vi "Hat Switch Interpreter.vi"(5 "Axis 6":dbl, 6 "Axis 5":dbl) -> (0 "Buttons":bool[](array[boolean]), 1 "Buttons Pressed":bool[](array[boolean]), 2 "Enum Status":T2(ring), 3 "Numeric Status":u8, 4 "Hat Switch Cluster":T1)   [LabVIEW 2013]
panel:
  # "ENUM LAYOUT"
  # "NUMERIC LAYOUT"
  # "North"
  # "1"
  # "Northeast"
  # "2"
  # "Northwest"
  # "8"
  # "West"
  # "East"
  # "7"
  # "3"
  # "Null"
  # "0"
  # "Southwest"
  # "Southeast"
  # "6"
  # "4"
  # "5"
  # "South"
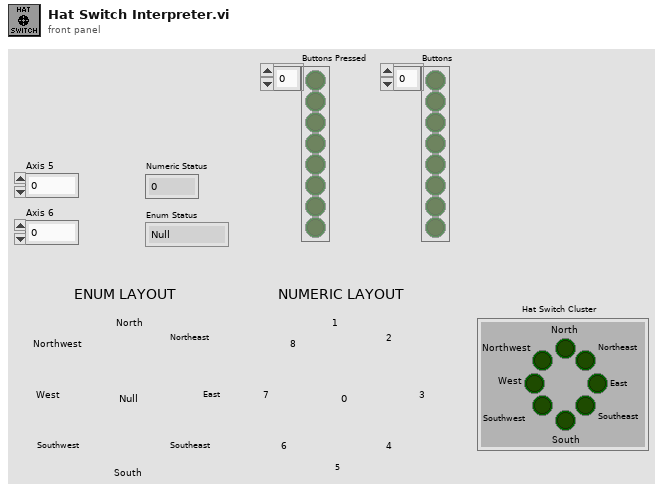
[diagram p1: front panel]
types:
  T1 = cluster{"North":bool, "Northeast":bool, "East":bool, "Southeast":bool, "South":bool, "Southwest":bool, "West":bool, "Northwest":bool}
  T2 = enum8{"Null", "North", "Northeast", "East", "Southeast", "South", "Southwest", "West", "Northwest"}
  T3 = cluster{"North":bool, "Northeast":bool, "East":bool, "Southeast":bool, "South":bool, "Northwest":bool, "Southwest":bool, "West":bool}
  T4 = cluster{"[0]":bool, "[1]":bool, "[2]":bool, "[3]":bool, "[4]":bool, "[5]":bool, "[6]":bool, "[7]":bool, "[8]":bool}
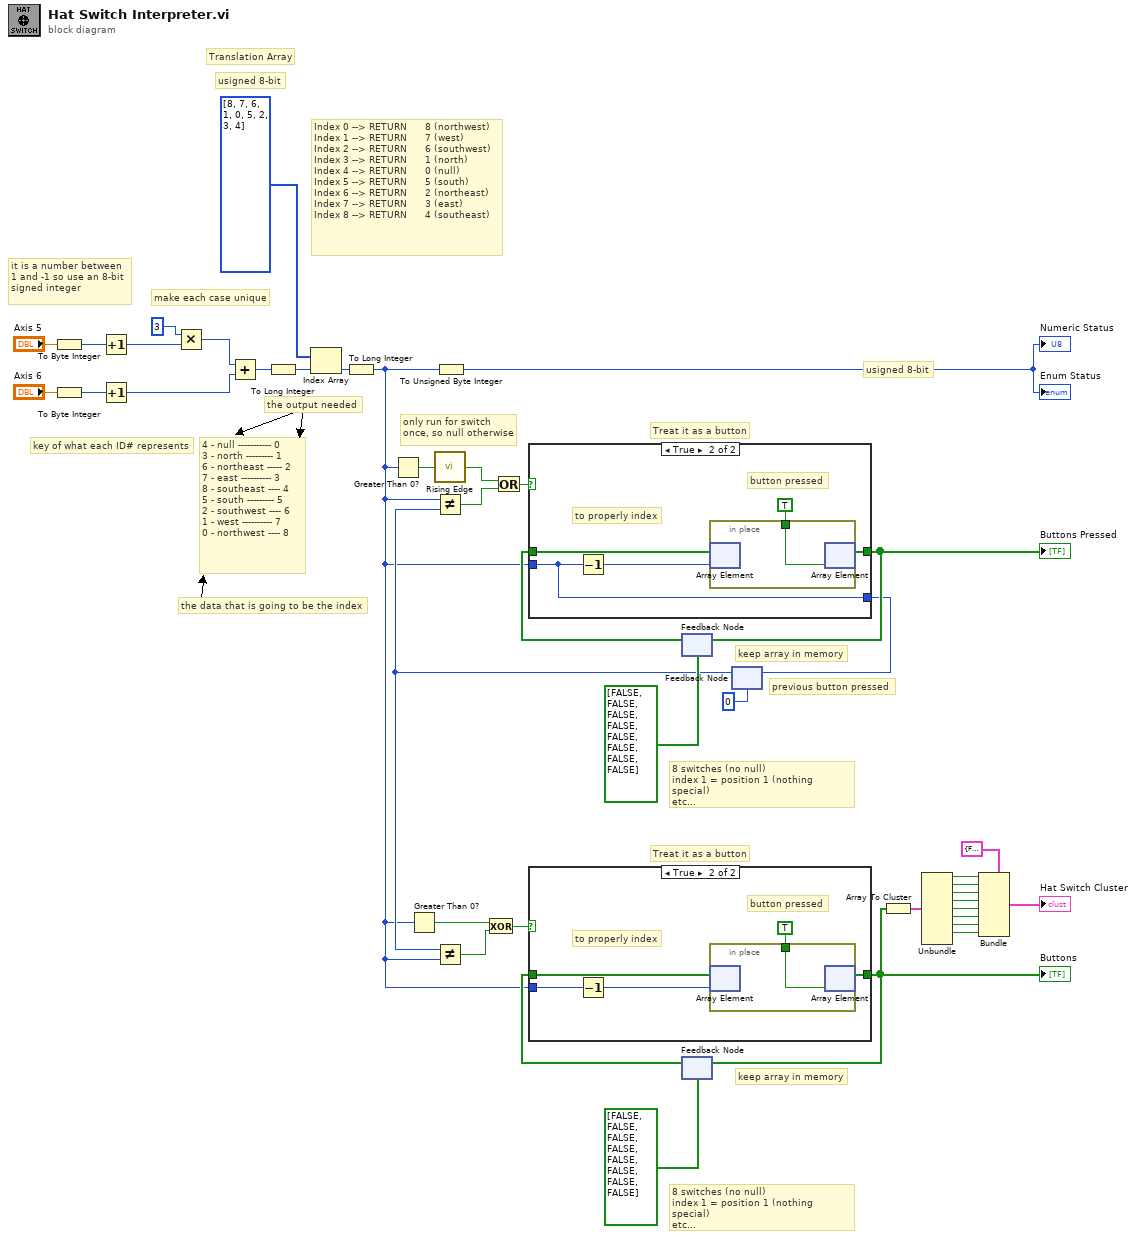
[diagram p0: block diagram]
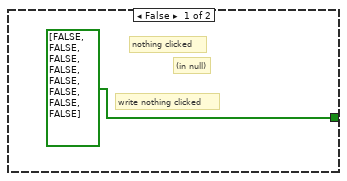
[diagram p2: hidden frame]
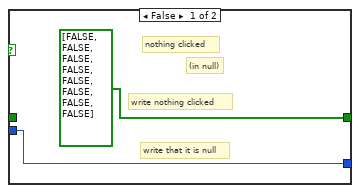
[diagram p3: hidden frame]
diagram:
  # "keep array in memory"
  # "8 switches (no null)\nindex 1 = position 1 (nothing special)\netc..."
  # "Treat it as a button"
  # "only run for switch\nonce, so null otherwise"
  # "keep array in memory"
  # "previous button pressed"
  # "8 switches (no null)\nindex 1 = position 1 (nothing special)\netc..."
  # "Treat it as a button"
  # "usigned 8-bit"
  # "the data that is going to be the index"
  # "the output needed"
  # "key of what each ID# represents"
  # "Index 0 --> RETURN      8 (northwest)\nIndex 1 --> RETURN      7 (west)\nIndex 2 --> RETURN      6 (southwest)\nIndex 3 --> RETURN      1 (north)\nIndex 4 --> RETURN      0 (null)\nIndex 5 --> RETURN      5 (south)\nIndex 6 --> RETURN      2 (northeast)\nIndex 7 --> RETURN      3 (east)\nIndex 8 --> RETURN      4 (southeast)"
  # "4 - null ----------- 0\n3 - north --------- 1\n6 - northeast ----- 2\n7 - east ---------- 3\n8 - southeast ---- 4\n5 - south --------- 5\n2 - southwest ---- 6\n1 - west ---------- 7\n0 - northwest ---- 8"
  # "Translation Array"
  # "usigned 8-bit"
  # "it is a number between\n1 and -1 so use an 8-bit\nsigned integer"
  # "make each case unique"
  n1 = To Byte Integer(number="Axis 5") -> (8bit integer=w35:i8)
  n2 = To Byte Integer(number="Axis 6") -> (8bit integer=w34:i8)
  n3 = Increment(x=w35) -> (x+1=w39:i8)
  n4 = Increment(x=w34) -> (x+1=w36:i8)
  n5 = Multiply(x=i8 3, y=w39) -> (x*y=w37:i8)
  n6 = Add(x=w37, y=w36) -> (x+y=w32:i8)
  n7 = To Long Integer(number=w32) -> (32bit integer=w31:i32)
  n8 = Index Array(array=u8[] [8, 7, 6, 1, 0, 5, 2, 3, 4], index=w31) -> (element=w22:u8)
  n9 = To Long Integer(number=w22) -> (32bit integer=w15:i32)
  n10 = Greater Than 0?(x=w15) -> (x > 0?=w25:bool)
  n11 = Greater Than 0?(x=w15) -> (x > 0?=w17:bool)
  n12 = call "Rising Edge.vi"("Input"=w25) -> ("Rising Edge"=w24:bool)
  n13 = To Unsigned Byte Integer(number=w15) -> (unsigned 8bit integer=→"Numeric Status" →"Enum Status":u8)
  n14 = feedback #1(bool[] [FALSE, FALSE, FALSE, FALSE, FALSE, FALSE, FALSE, FALSE]) -> (w29:bool[])
  n15 = feedback #2(bool[] [FALSE, FALSE, FALSE, FALSE, FALSE, FALSE, FALSE, FALSE]) -> (w19:bool[])
  n16 = feedback #3(0) -> (w16:i32)
  n17 = Not Equal?(x=w15, y=w16) -> (x != y?=w21:bool)
  n18 = Not Equal?(x=w16, y=w15) -> (x != y?=w13:bool)
  n19 = Exclusive Or(1:w13, 2:w17) -> (0:w14:bool)
  n20 = Or(x=w24, y=w21) -> (x .or. y?=w23:bool)
  n21 = case shown="True" w23 {
    tunnel: w29 -> [_ w48]
    tunnel: [bool[] [FALSE, FALSE, FALSE, FALSE, FALSE, FALSE, FALSE, FALSE] w47] -> w28
    tunnel: w15 -> [w43 w44]
    tunnel: [w43 w44] -> w26
    frame False {
      # "write nothing clicked"
      # "write that it is null"
      # "(in null)"
      # "nothing clicked"
    }
    frame True {
      # "to properly index"
      # "button pressed"
      n22 = Decrement(x=w44) -> (x-1=w45:i32)
      n23 = in-place {
        in-place-border: TRUE -> [w49]
        n24 = in-place-array #4(w48, w45) -> ()  [unwired: 1 out]
        n25 = in-place-array #4(w49) -> (w47:bool[])  [unwired: 1 out]
      }
    }
  }
  "Buttons Pressed" <- w28
  n26 = case shown="True" w14 {
    tunnel: w19 -> [_ w55]
    tunnel: [bool[] [FALSE, FALSE, FALSE, FALSE, FALSE, FALSE, FALSE, FALSE] w54] -> w12
    tunnel: w15 -> [_ w51]
    frame False {
      # "write nothing clicked"
      # "(in null)"
      # "nothing clicked"
    }
    frame True {
      # "to properly index"
      # "button pressed"
      n27 = Decrement(x=w51) -> (x-1=w52:i32)
      n28 = in-place {
        in-place-border: TRUE -> [w56]
        n29 = in-place-array #5(w55, w52) -> ()  [unwired: 1 out]
        n30 = in-place-array #5(w56) -> (w54:bool[])  [unwired: 1 out]
      }
    }
  }
  "Buttons" <- w12
  n31 = feedback-in #1(w28) -> ()
  n32 = feedback-in #2(w12) -> ()
  n33 = feedback-in #3(w26) -> ()
  n34 = Array To Cluster(array=w12) -> (cluster=w11:T4)
  n35 = Unbundle(w11) -> ("[0]"=w9:bool, "[1]"=w1:bool, "[2]"=w2:bool, "[3]"=w3:bool, "[4]"=w4:bool, "[5]"=w5:bool, "[6]"=w6:bool, "[7]"=w7:bool)  [unwired: 1 out]
  n36 = Bundle(cluster=T3 {"North"=FALSE, "Northeast"=FALSE, "East"=FALSE, "Southeast"=FALSE, "South"=FALSE, "Northwest"=FALSE, "Southwest"=FALSE, "West"=FALSE} ("Hat Switch Cluster"), "North"=w9, "Northeast"=w1, "East"=w2, "Southeast"=w3, "South"=w4, "Northwest"=w5, "Southwest"=w6, "West"=w7) -> (→"Hat Switch Cluster":T3)
